vi "date_time_string.vi"() -> (0 "date/time string":string)   [LabVIEW 2018]
panel:
  in  "time format string (%c)":string="%Y%m%d_%H%M"
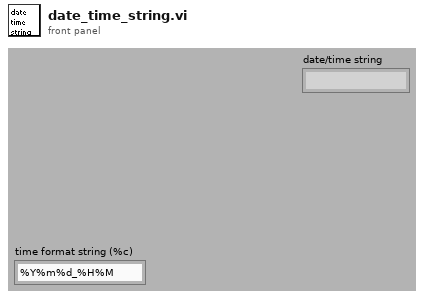
[diagram p1: front panel]
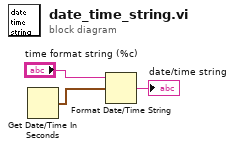
[diagram p0: block diagram]
diagram:
  n1 = Get Date/Time In Seconds() -> (seconds since 1Jan1904=w1:timestamp)
  n2 = Format Date/Time String(time format string (%c)="time format string (%c)", seconds (now)=w1) -> (date/time string=→"date/time string":string)  [unwired: 1 in]
